vi "Curtin1_Color 2.vi"(8 "Offset":u16, 10 "Files in":T1[](array[typedef])) -> (2 "New color":u32)   [LabVIEW 2024]
uses:
  Curtin1_Label.ctl
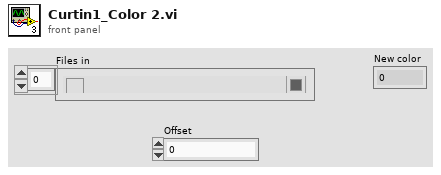
[diagram p1: front panel]
types:
  T1 = typedef "Curtin1_Label.ctl" = cluster{"Show?":bool, "Name":string, "Color":u32, "Path":path, "Show Notes":bool}
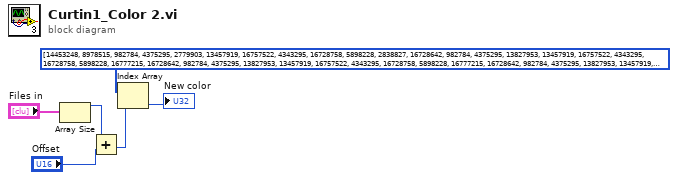
[diagram p0: block diagram]
diagram:
  n1 = Array Size(array="Files in") -> (size(s)=w2:i32)
  n2 = Add(x=w2, y="Offset") -> (x+y=w1:i32)
  n3 = Index Array(array=u32[] [14453248, 8978515, 982784, 4375295, 2779903, 13457919, 16757522, 4343295, 16728758, 5898228, 2838827, 16728642, 982784, 4375295, 13827953, 13457919, 16757522, 4343295, 16728758, 5898228, 16777215, 16728642, 982784, 4375295, 13827953, 13457919, 16757522, 4343295, 16728758, 5898228, 16777215, 16728642, 982784, 4375295, 13827953, 13457919, 16757522, 4343295, 16728758, 5898228, 16777215, 16728642, 982784, 4375295, 13827953, 13457919, 16757522, 4343295, 16728758, 5898228, 16777215, 16728642, 982784, 4375295, 13827953, 13457919, 16757522, 4343295, 16728758, 5898228, 16777215, 16728642, 982784, 4375295, 13827953, 13457919, 16757522, 4343295, 16728758, 5898228, 16777215, 16728642, 982784, 4375295, 13827953, 13457919, 16757522, 4343295, 16728758, 5898228, 16777215, 16728642, 982784, 4375295, 13827953, 13457919, 16757522, 4343295, 16728758, 5898228, 16777215, 16728642, 982784, 4375295, 13827953, 13457919, 16757522, 4343295, 16728758, 5898228] ("Array"), index=w1) -> (element=→"New color":u32)
